vi "DirectorState.vi"(0 "内部故障":cluster{"模拟故障？":bool, "数字故障？":bool}, 1 "外部故障":bool, 2 "电源状态":T1, 3 "触发状态":bool, 4 "计算模块状态":bool, 5 "READY_COLD_TO_HOT":bool) -> (16 "电源下一个状态":T1, 19 "enable":bool)   [LabVIEW 2018]
uses:
  Ctl/State.ctl
panel:
  in  "内部故障":bool
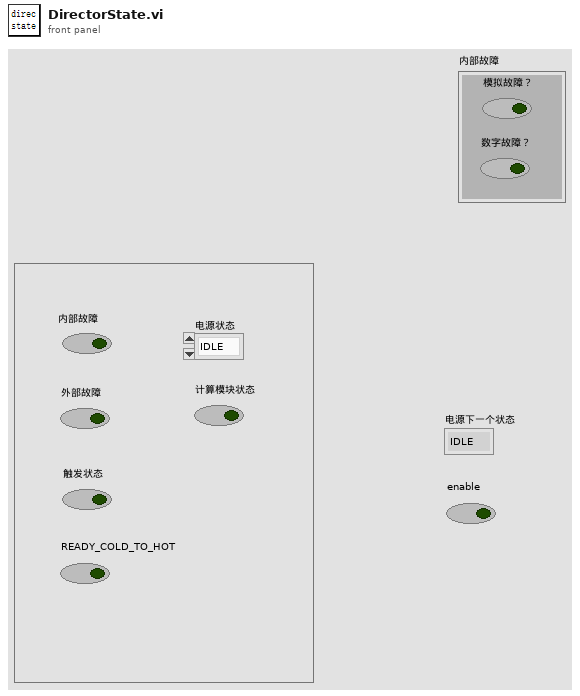
[diagram p1: front panel]
types:
  T1 = typedef "State.ctl" = enum16{"IDLE", "READY_COLD", "READY_HOT", "RUN", "ERROR"}
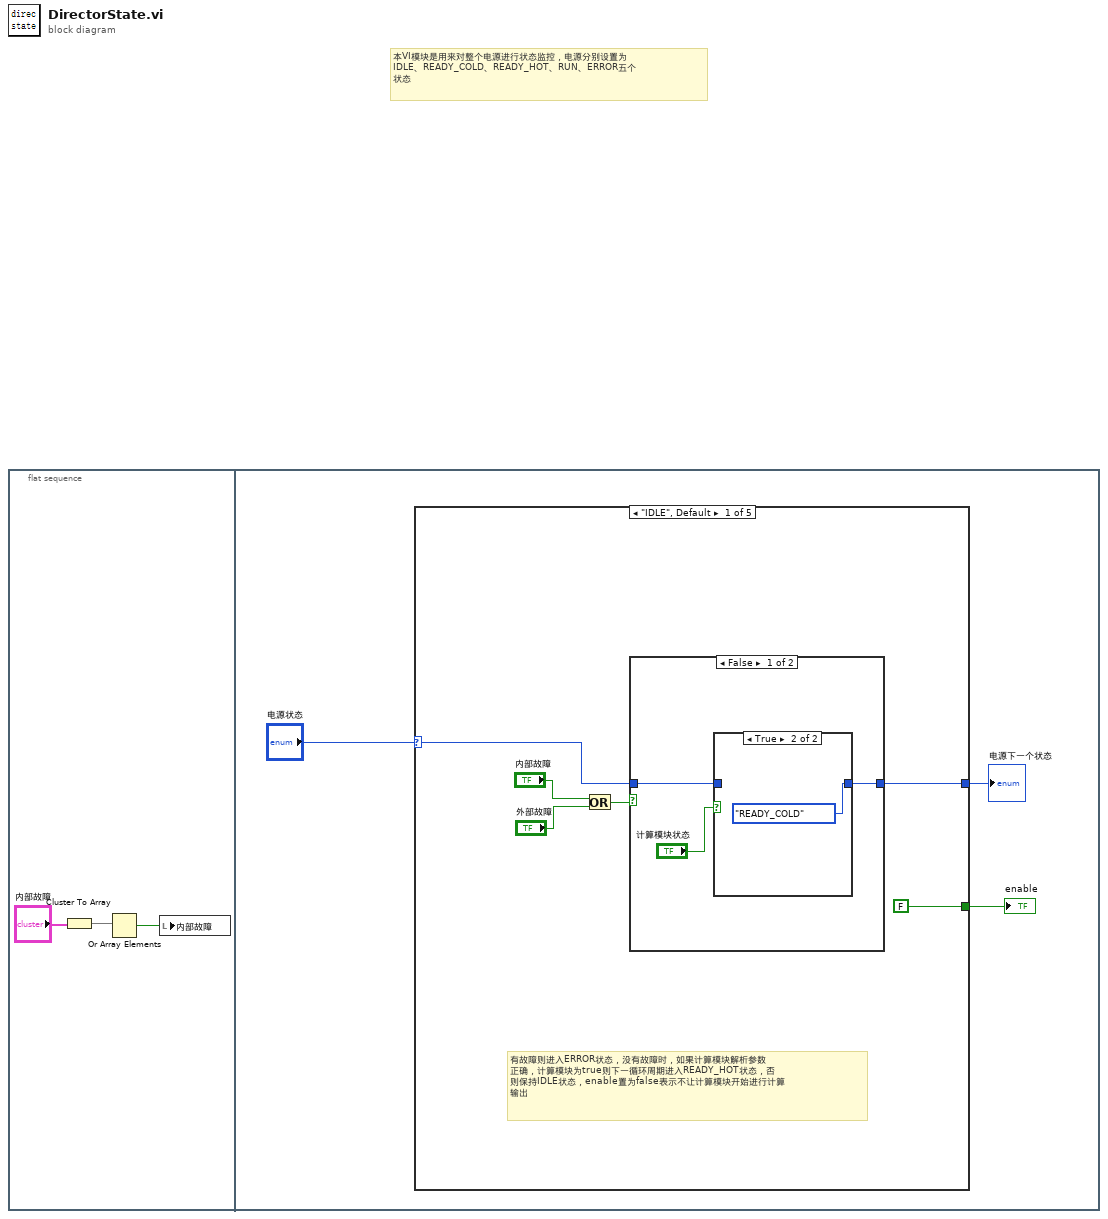
[diagram p0: block diagram]
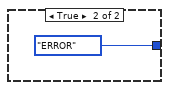
[diagram p3: hidden frame]
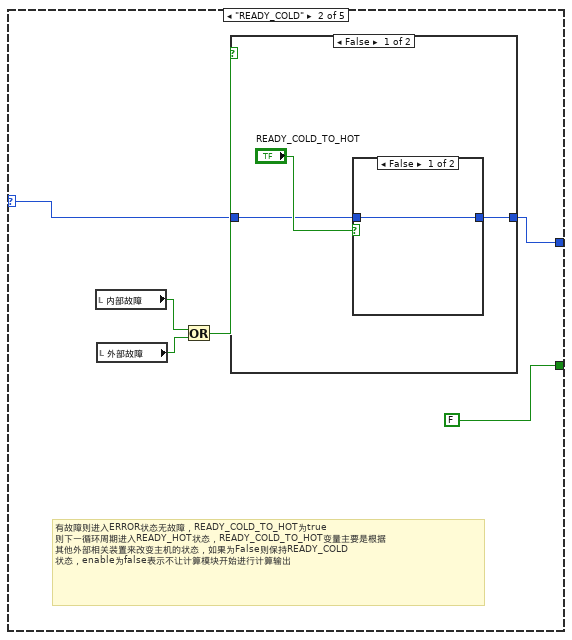
[diagram p4: hidden frame]
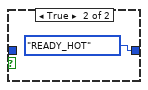
[diagram p5: hidden frame]
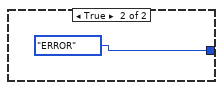
[diagram p6: hidden frame]
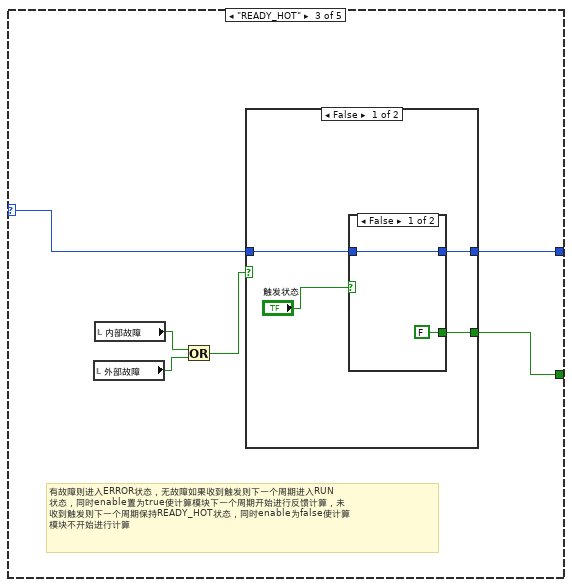
[diagram p7: hidden frame]
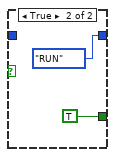
[diagram p8: hidden frame]
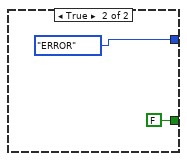
[diagram p9: hidden frame]
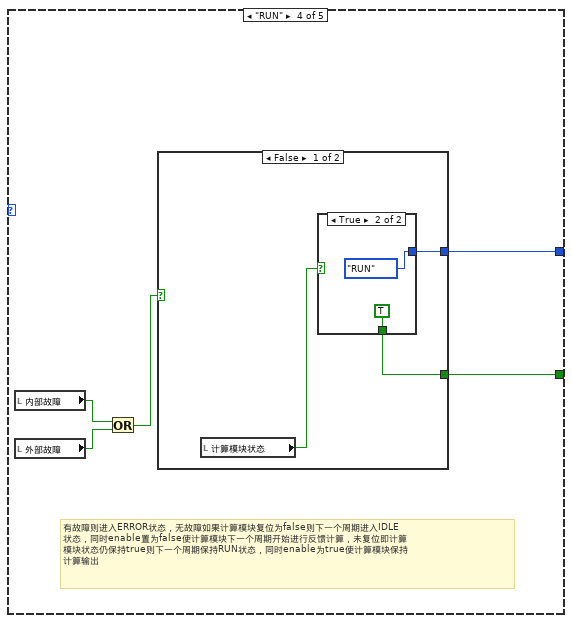
[diagram p10: hidden frame]
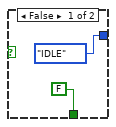
[diagram p11: hidden frame]
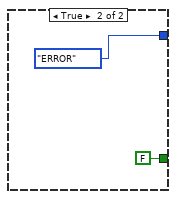
[diagram p12: hidden frame]
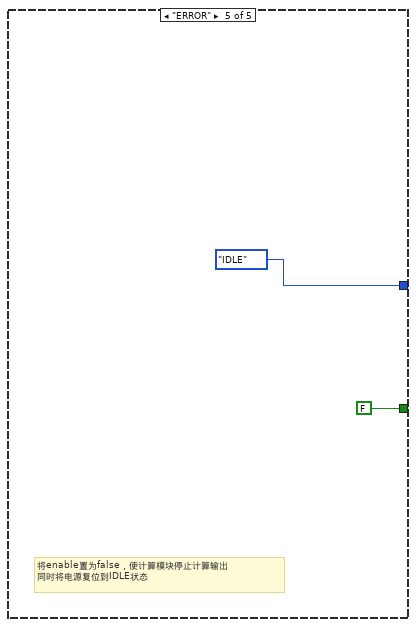
[diagram p13: hidden frame]
diagram:
  # "本VI模块是用来对整个电源进行状态监控，电源分别设置为\nIDLE、READY_COLD、READY_HOT、RUN、ERROR五个\n状态"
  n1 = flat-sequence {
    frame #0 {
      n2 = Cluster To Array(cluster="内部故障") -> (array=w2:bool[])
      n3 = Or Array Elements(Boolean array=w2) -> (logical OR=w3:bool)
      n4 = local write "内部故障"(w3) -> ()
    }
    frame #1 {
      n5 = case shown="\"IDLE\", Default" "电源状态" {
        selector: "电源状态" -> [w8 w20 w32 _ _]
        tunnel: [w9 w21 w33 w48 State."IDLE" ("枚举")] -> w5
        tunnel: [FALSE FALSE w31 w47 FALSE] -> w4
        frame "IDLE", Default {
          # "有故障则进入ERROR状态，没有故障时，如果计算模块解析参数\n正确，计算模块为true则下一循环周期进入READY_HOT状态，否\n则保持IDLE状态，enable置为false表示不让计算模块开始进行计算\n输出"
          n6 = Or(x="内部故障", y="外部故障") -> (x .or. y?=w10:bool)
          n7 = case shown="False" w10 {
            tunnel: [w14 State."ERROR" ("枚举")] -> w9
            tunnel: w8 -> [w13 _]
            frame False {
              n8 = case shown="True" "计算模块状态" {
                tunnel: [w16 State."READY_COLD" ("枚举")] -> w14
                tunnel: w13 -> [w16 _]
                frame False {
                }
                frame True {
                }
              }
            }
            frame True {
            }
          }
        }
        frame "READY_COLD" {
          # "有故障则进入ERROR状态无故障，READY_COLD_TO_HOT为true\n则下一循环周期进入READY_HOT状态，READY_COLD_TO_HOT变量主要是根据\n其他外部相关装置来改变主机的状态，如果为False则保持READY_COLD\n状态，enable为false表示不让计算模块开始进行计算输出"
          n9 = local read "内部故障"() -> (w24:bool)
          n10 = local read "外部故障"() -> (w23:bool)
          n11 = Or(x=w24, y=w23) -> (x .or. y?=w22:bool)
          n12 = case shown="False" w22 {
            tunnel: [w26 State."ERROR" ("枚举")] -> w21
            tunnel: w20 -> [w25 _]
            frame False {
              n13 = case shown="False" "READY_COLD_TO_HOT" {
                tunnel: [w28 State."READY_HOT" ("枚举")] -> w26
                tunnel: w25 -> [w28 _]
                frame False {
                }
                frame True {
                }
              }
            }
            frame True {
            }
          }
        }
        frame "READY_HOT" {
          # "有故障则进入ERROR状态，无故障如果收到触发则下一个周期进入RUN\n状态，同时enable置为true使计算模块下一个周期开始进行反馈计算，未\n收到触发则下一个周期保持READY_HOT状态，同时enable为false使计算\n模块不开始进行计算"
          n14 = local read "外部故障"() -> (w35:bool)
          n15 = local read "内部故障"() -> (w36:bool)
          n16 = Or(x=w36, y=w35) -> (x .or. y?=w34:bool)
          n17 = case shown="False" w34 {
            tunnel: [w39 State."ERROR" ("枚举")] -> w33
            tunnel: w32 -> [w38 _]
            tunnel: [w37 FALSE] -> w31
            frame False {
              n18 = case shown="False" "触发状态" {
                tunnel: [w42 State."RUN" ("枚举")] -> w39
                tunnel: w38 -> [w42 _]
                tunnel: [FALSE TRUE] -> w37
                frame False {
                }
                frame True {
                }
              }
            }
            frame True {
            }
          }
        }
        frame "RUN" {
          # "有故障则进入ERROR状态，无故障如果计算模块复位为false则下一个周期进入IDLE\n状态，同时enable置为false使计算模块下一个周期开始进行反馈计算，未复位即计算\n模块状态仍保持true则下一个周期保持RUN状态，同时enable为true使计算模块保持\n计算输出"
          n19 = local read "内部故障"() -> (w51:bool)
          n20 = local read "外部故障"() -> (w50:bool)
          n21 = Or(x=w51, y=w50) -> (x .or. y?=w49:bool)
          n22 = case shown="False" w49 {
            tunnel: [w53 State."ERROR" ("枚举")] -> w48
            tunnel: [w52 FALSE] -> w47
            frame False {
              n23 = local read "计算模块状态"() -> (w54:bool)
              n24 = case shown="True" w54 {
                tunnel: [State."IDLE" ("枚举") State."RUN" ("枚举")] -> w53
                tunnel: [FALSE TRUE] -> w52
                frame False {
                }
                frame True {
                }
              }
            }
            frame True {
            }
          }
        }
        frame "ERROR" {
          # "将enable置为false，使计算模块停止计算输出\n同时将电源复位到IDLE状态"
        }
      }
      "enable" <- w4
      "电源下一个状态" <- w5
    }
  }
